vi "AppendVeloc.vi"(4 "GroupSize":i32, 6 "PrimeiroCanal":i32=1, 7 "MaxFreq":dbl=200.0, 8 "error in":errorcluster, 9 "VelocTimeStamps":timestamp[](array[timestamp]), 10 "MaxVelocs":dbl[](array[numeric]), 11 "DirPath":path) -> (0 "error out":errorcluster, 3 "Texto":string)   [LabVIEW 2016]
uses:
  DataForPython/DataPython.ctl
  <vilib>/Analysis/baseanly.llb/Mean (DBL).vi
  <vilib>/addons/Digital Filter Design/Design.llb/DFD IIR Notch Peak Design by BW.vi
  <vilib>/addons/Digital Filter Design/Process.llb/DFD Filtering (Array NChan).vi
  <vilib>/Analysis/NI_AALPro.lvlib
  <vilib>/addons/Digital Filter Design/NI_DigFilterLicensed.lvlib
  <vilib>/Analysis/NI_AALBase.lvlib
panel:
  out "input":T1[][](array[typedef])
  out "Data":T1[][](array[typedef])
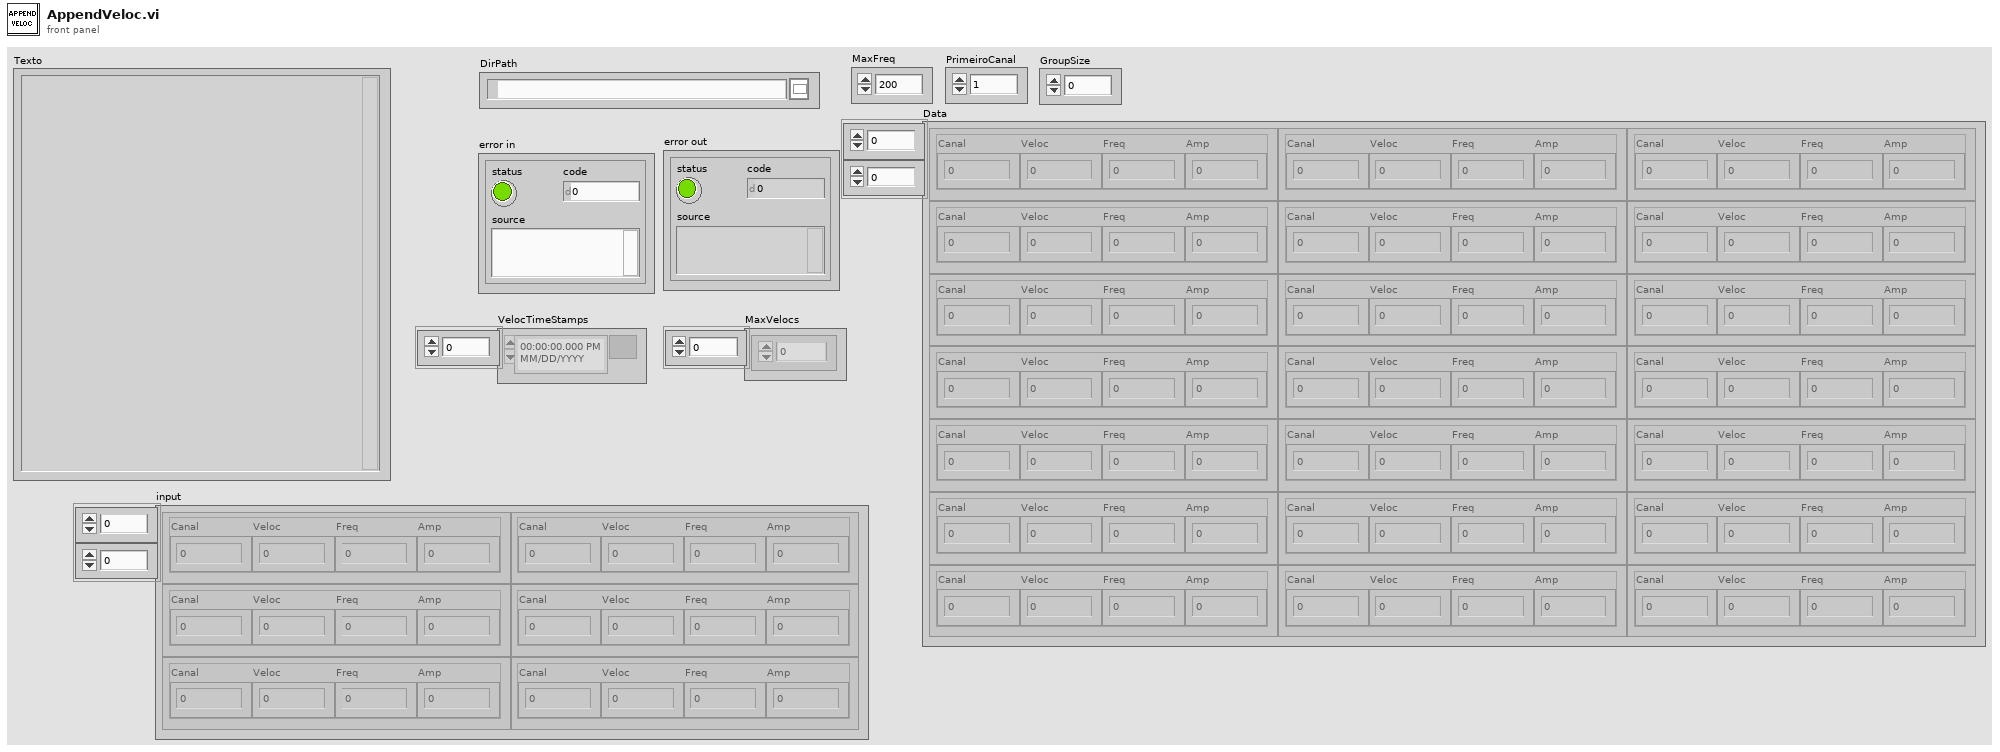
[diagram p1: front panel]
types:
  T1 = typedef "DataPython.ctl" = cluster{"Canal":i32, "Veloc":dbl, "Freq":dbl, "Amp":dbl}
  T2 = typedef "NI_DigFilterLicensed.lvlib/DFD Filter Obj.ctl" = cluster{"mSRate_Fs":dbl, "mSRate_Version":string, "mSRate_Comments":string, "mSRate_OrgCoef":T3, "mSRate_CurCoef":T3, "mSRate_Quantized?":bool, "mSRate_QCoef":T3, "mSRate_QSettings":T5[], "mSRate_Order":i32, "mSRate_Scaling":cluster{"mSRate_ScaleByPowerOf2?":bool, "mSRate_ScaleType":T7}}
  T3 = typedef "NI_DigFilterLicensed.lvlib/DFD Filter Coef.ctl" = cluster{"type":T4, "gain":dbl, "coef a (k)":dbl[], "coef b (v)":dbl[]}
  T4 = typedef "NI_DigFilterLicensed.lvlib/DFD Filter Structure Type Selector.ctl" = enum16{"Undefined", "FIR Direct Form", "FIR Direct Form Transposed", "FIR Symmetric", "FIR Antisymmetric", "IIR Direct Form I", "IIR Direct Form I Transposed", "IIR Direct Form II", "IIR Direct Form II Transposed", "IIR Cascaded Second Order Sections Form I", "IIR Cascaded Second Order Sections Form I Transposed", "IIR Cascaded Second Order Sections Form II", "IIR Cascaded Second Order Sections Form II Transposed", "Lattice Allpass (basic sections)", "Lattice Allpass (one multiplier sections)", "Lattice Allpass (normalized sections)", "Lattice AR (basic sections)", "Lattice AR (one multiplier sections)", "Lattice AR (normalized sections)", "Lattice MA (minimum phase)", "Lattice MA (maximum phase)", "Lattice ARMA (basic sections)", "Lattice ARMA (one multiplier sections)", "Lattice ARMA (normalized sections)"}
  T5 = typedef "NI_DigFilterLicensed.lvlib/dfd_Internal Quantization Settings.ctl" = cluster{"source":T6, "wl":i16, "iwl":i16, "overflow mode":enum16{"Saturation", "Wrap"}, "rounding mode":enum16{"Nearest", "Truncation"}, "signed?":bool}
  T6 = typedef "NI_DigFilterLicensed.lvlib/dfd_Internal Quantization Srcs.ctl" = u16
  T7 = typedef "NI_DigFilterLicensed.lvlib/DFD Coef Norm Type.ctl" = enum16{"No Norm", "Time Domain 1-Norm", "Time Domain 2-Norm", "Time Domain Inf-Norm"}
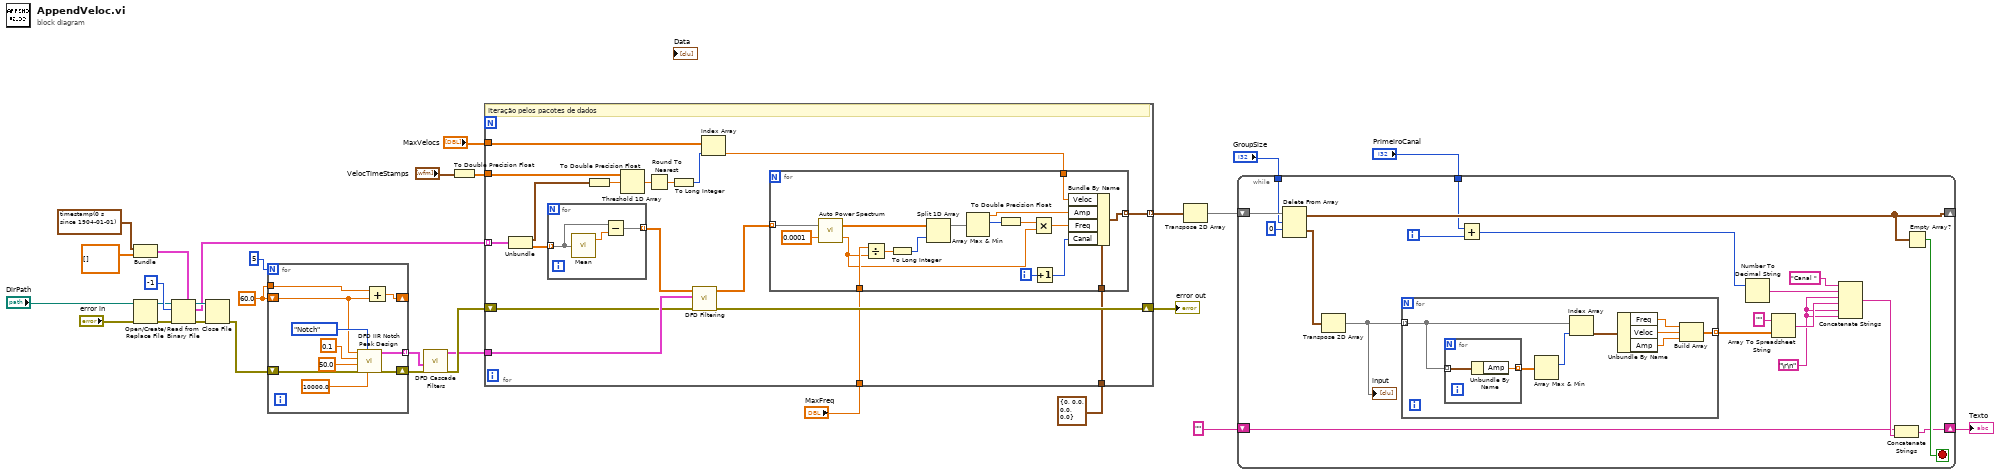
[diagram p0: block diagram]
diagram:
  w19 = 60.0 ("f0 [Hz]")
  n1 = Bundle(timestamp(0 s since 1904-01-01), dbl[][] []) -> (w30:cluster{timestamp, dbl[][]})  [unwired: 1 in]
  n2 = Open/Create/Replace File(file path (use dialog)="DirPath", error in="error in") -> (refnum out=w23:refnum<file>, error out=w24:errorcluster)  [unwired: 4 in, 1 out]
  n3 = Read from Binary File(5:w30, 8:w24, 10:-1 ("count (1)"), 11:w23) -> (0:w27:errorcluster, 2:w12:cluster{timestamp, dbl[][]}[], 3:w26:refnum<file>)  [unwired: 2 in, 1 out]
  n4 = Close File(refnum=w26, error in=w27) -> (error out=w18:errorcluster)  [unwired: 1 out]
  n5 = for {
    N: 5 -> [_]
    tunnel: [w37] -> w17 mode=indexing
    shift-right: [w34] -> _
    shift-left: w19 -> [w33]
    tunnel: w19 -> [w35]
    shift-right: [w31] -> w16
    shift-left: w18 -> [w32]
    n6 = call-poly <vilib>:"DFD IIR Notch Peak Design.vi"("fs [Hz]"=10000.0, "filter type"=enum16{"Notch", "Peak"}."Notch", "error in (no error)"=w32, "Ab [dB]"=50.0, "Df [Hz]"=0.1, "f0 [Hz]"=w33) -> ("error out"=w31:errorcluster, "filter out"=w37:T2)  [unwired: 4 in]
    n7 = Add(x=w35, y=w33) -> (x+y=w34:dbl)
  }
  n8 = call <vilib>:"DFD Cascade Filters.vi"("error in (no error)"=w16, "filters in"=w17) -> ("error out"=w15:errorcluster, "filter out"=w14:T2)  [unwired: 8 in]
  n9 = To Double Precision Float(number="VelocTimeStamps") -> (double precision float=w8:dbl[])
  n10 = for {
    tunnel: w12 -> [w58] mode=indexing
    tunnel: w14 -> [w57]
    shift-right: [w52] -> w13
    shift-left: w15 -> [w56]
    tunnel: "MaxFreq" -> [w51]
    tunnel: T1 {"Canal"=0, "Veloc"=0.0, "Freq"=0.0, "Amp"=0.0} ("DataPython") -> [w50]
    tunnel: w8 -> [w44]
    tunnel: "MaxVelocs" -> [w43]
    tunnel: [w41] -> w4 mode=indexing
    # "Iteração pelos pacotes de dados"
    n11 = Unbundle(w58) -> (w45:timestamp, w54:dbl[][])
    n12 = for {
      tunnel: w54 -> [w60] mode=indexing
      tunnel: [w59] -> w53 mode=indexing
      n13 = call-poly <vilib>:"Mean.vi"("X"=w60) -> ("mean"=w61:dbl)  [unwired: 1 out]
      n14 = Subtract(x=w60, y=w61) -> (x-y=w59:dbl[])
    }
    n15 = To Double Precision Float(number=w45) -> (double precision float=w46:dbl)
    n16 = Threshold 1D Array(2:w46, 3:w44) -> (0:w47:dbl)  [unwired: 1 in]
    n17 = Round To Nearest(number=w47) -> (nearest integer value=w48:dbl)
    n18 = To Long Integer(number=w48) -> (32bit integer=w49:i32)
    n19 = call-poly <vilib>:"DFD Filtering.vi"("error in (no error)"=w56, "filter"=w57, "signal in"=w53) -> ("error out"=w52:errorcluster, "signal out"=w55:dbl[][])  [unwired: 7 in]
    n20 = Index Array(array=w43, index=w49) -> (element=w42:dbl)
    n21 = for {
      tunnel: w55 -> [w78] mode=indexing
      tunnel: w51 -> [w76]
      tunnel: w50 -> [w68]
      tunnel: w42 -> [w65]
      tunnel: [w64] -> w41 mode=indexing
      i -> [w63]
      n22 = call <vilib>:"Auto Power Spectrum.vi"("dt"=0.0001, "Signal (V)"=w78) -> ("df"=w69:dbl, "Power Spectrum (V^2 rms)"=w75:dbl[])
      n23 = Divide(x=w76, y=w69) -> (x/y=w74:dbl)
      n24 = To Long Integer(number=w74) -> (32bit integer=w73:i32)
      n25 = Split 1D Array(array=w75, index=w73) -> (first subarray=w72:dbl[])  [unwired: 1 out]
      n26 = Array Max & Min(array=w72) -> (max value=w66:dbl, max index (indices)=w71:i32)  [unwired: 2 out]
      n27 = To Double Precision Float(number=w71) -> (double precision float=w70:dbl)
      n28 = Multiply(x=w70, y=w69) -> (x*y=w67:dbl)
      n29 = Increment(x=w63) -> (x+1=w62:i32)
      n30 = Bundle By Name(cluster=w68, "Veloc"=w65, "Amp"=w66, "Freq"=w67, "Canal"=w62) -> (w64:T1)
    }
  }
  "error out" <- w13
  n31 = Transpose 2D Array(2D array=w4) -> (transposed array=w3:T1[][])
  n32 = while {
    shift-right: [w94] -> _
    shift-left: w3 -> [w97]
    tunnel: "GroupSize" -> [w96]
    tunnel: "PrimeiroCanal" -> [w91]
    shift-right: [w79] -> w1
    shift-left: "" -> [w80]
    i -> [w92]
    stop <- w93 stop-if-true
    w82 = "\r\n"
    n33 = Delete From Array(array=w97, length=w96, index (row)=0) -> (deleted portion=w90:T1[][], array with subset deleted=w94:T1[][])  [unwired: 1 in]
    n34 = Transpose 2D Array(2D array=w90) -> (transposed array=w89:T1[][])
    "input" <- w89
    n35 = for {
      tunnel: w89 -> [w104] mode=indexing
      tunnel: [w98] -> w88 mode=indexing
      n36 = for {
        tunnel: w104 -> [w107] mode=indexing
        tunnel: [w106] -> w105 mode=indexing
        n37 = Unbundle By Name(w107) -> ("Amp"=w106:dbl)
      }
      n38 = Array Max & Min(array=w105) -> (max index (indices)=w103:i32)  [unwired: 3 out]
      n39 = Index Array(array=w104, index=w103) -> (element=w99:T1)
      n40 = Unbundle By Name(w99) -> ("Freq"=w100:dbl, "Veloc"=w101:dbl, "Amp"=w102:dbl)
      n41 = Build Array(w100, w101, w102) -> (w98:dbl[])
    }
    n42 = Add(x=w91, y=w92) -> (x+y=w81:i32)
    n43 = Number To Decimal String(number=w81) -> (decimal integer string=w86:string)  [unwired: 1 in]
    n44 = Array To Spreadsheet String(array=w88, 3:"" ("format string")) -> (spreadsheet string=w85:string)  [unwired: 1 in]
    n45 = Concatenate Strings("Canal " ("string"), w86, w82, w85, w82, w82) -> (w83:string)
    n46 = Concatenate Strings(w80, w83) -> (w79:string)
    n47 = Empty Array?(array=w94) -> (empty?=w93:bool)
  }
  "Texto" <- w1
